vi "Read Multi Eval Meas EVM Results.vi"(8 "error in (no error)":errorcluster, 9 "Result Type (Current)":i32(ring) items=["Current"=0, "Average"=1, "Maximum"=4], 10 "Instance (1)":T1=1, 11 "VISA resource name":refnum<visa-resource-name>) -> (0 "error out":errorcluster, 1 "EVM Results":cluster{"Low":dbl, "High":dbl}[](array[cluster]) {"High" format="%^.3e"; "Low" format="%^.3e"}, 2 "Reliability":i32, 3 "VISA resource name out":refnum<visa-resource-name>)   [LabVIEW 2020, in "Rohde&Schwarz CMXP NR FR2 Measurement.lvlib"]
doc: "Starts a new single shot measurement and returns the multi eval measurement EVM results.\n\nAttributes:\nRSCMXPNRFR2M_ATTR_READ_MULTI_EVAL_MEASUREMENT_EVM_AVERAGE_RESULTS\nRSCMXPNRFR2M_ATTR_READ_MULTI_EVAL_MEASUREMENT_EVM_CURRENT_RESULTS\nRSCMXPNRFR2M_ATTR_READ_MULTI_EVAL_MEASUREMENT_EVM_MAXIMUM_RESULTS\n\nRemote-control commands:\nREAD:NRMMw:MEAS<i>:MEValuation:EVMagnitude:AVERage?\nREAD:NRMMw:MEAS<i>:MEValuation:EVMagnitude:CURRent?\nREAD:NRMMw:MEAS<i>:MEValuation:EVMagnitude:MAXimum?"
uses:
  <instrlib>/Rohde&Schwarz CMXP NR FR2 Measurement/Rohde&Schwarz CMXP NR FR2 Measurement.lvlib
  <instrlib>/Rohde&Schwarz CMXP NR FR2 Measurement/Private/_Instance.ctl
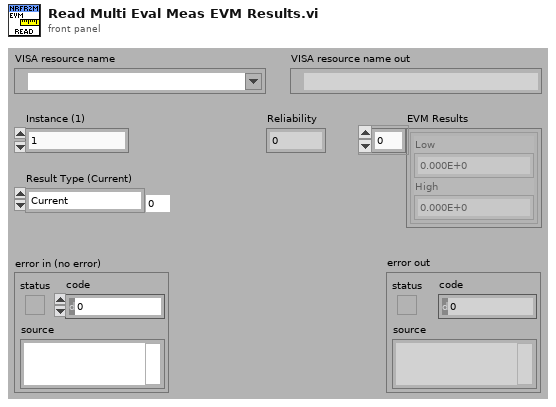
[diagram p1: front panel]
types:
  T1 = typedef "Rohde&Schwarz CMXP NR FR2 Measurement.lvlib/_Instance.ctl" = i32
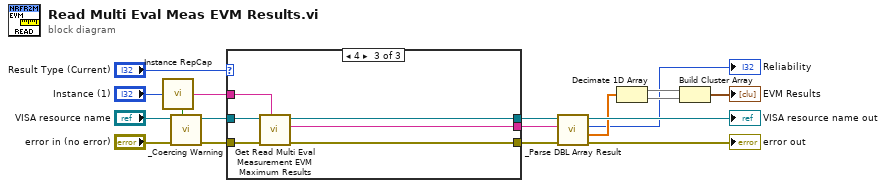
[diagram p0: block diagram]
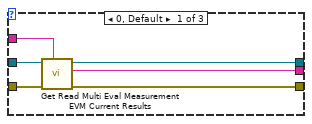
[diagram p2: hidden frame]
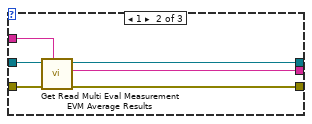
[diagram p3: hidden frame]
diagram:
  n1 = call <instrlib>:"Instance RepCap.vi"("Instance In"="Instance (1)") -> ("In Range?"=w5:bool, "RepCap Identifier Out"=w18:string)  [unwired: 1 in]
  n2 = call <instrlib>:"_Coercing Warning.vi"("In Range?"=w5, "error in (no error)"="error in (no error)", "VISA resource name"="VISA resource name") -> ("error out"=w3:errorcluster, "VISA resource name out"=w4:refnum<visa-resource-name>)  [unwired: 7 in]
  n3 = case shown="4" "Result Type (Current)" {
    tunnel: w3 -> [w22 w30 w36]
    tunnel: w4 -> [w21 w29 w35]
    tunnel: [w20 w28 w34] -> w16
    tunnel: [w19 w27 w33] -> w15
    tunnel: w18 -> [w24 w26 w32]
    tunnel: [w23 w25 w31] -> w12
    frame 0, Default {
      n4 = call "Get Read Multi Eval Measurement EVM Current Results"("Repeated Capabilities"=w24, "error in (no error)"=w22, "instrument handle"=w21) -> ("error out"=w20:errorcluster, "Read Multi Eval Measurement EVM Current Results"=w23:string, "instrument handle out"=w19:refnum<visa-resource-name>)  [unwired: 6 in]
    }
    frame 1 {
      n5 = call "Get Read Multi Eval Measurement EVM Average Results"("Repeated Capabilities"=w26, "error in (no error)"=w30, "instrument handle"=w29) -> ("error out"=w28:errorcluster, "Read Multi Eval Measurement EVM Average Results"=w25:string, "instrument handle out"=w27:refnum<visa-resource-name>)  [unwired: 6 in]
    }
    frame 4 {
      n6 = call "Get Read Multi Eval Measurement EVM Maximum Results"("Repeated Capabilities"=w32, "error in (no error)"=w36, "instrument handle"=w35) -> ("error out"=w34:errorcluster, "Read Multi Eval Measurement EVM Maximum Results"=w31:string, "instrument handle out"=w33:refnum<visa-resource-name>)  [unwired: 6 in]
    }
  }
  n7 = call <instrlib>:"_Parse DBL Array Result.vi"("error in (no error)"=w16, "Input String"=w12, "VISA resource name"=w15) -> ("error out"=→"error out":errorcluster, "Results"=w11:dbl[], "Reliability"=→"Reliability":i32, "VISA resource name out"=→"VISA resource name out":refnum<visa-resource-name>)  [unwired: 5 in]
  n8 = Decimate 1D Array(w11) -> (w10:dbl[], w9:dbl[])
  n9 = Build Cluster Array ("Index & Bundle Cluster Array")(w10, w9) -> (→"EVM Results":cluster{"Element":dbl, "Element":dbl}[])
